vi "Check Condition.vi"(8 "error in (no error)":errorcluster, 11 "InterlockControl in":refnum<class "InterlockControl.lvclass">) -> (0 "error out":errorcluster, 2 "Interlocked":bool, 3 "InterlockControl out":refnum<class "InterlockControl.lvclass">)   [LabVIEW 2020, in "VolatusControl.lvlib" / "InterlockControl.lvclass"]
uses:
  InterlockControl.lvclass
  InterlockControl.lvclass/InterlockControl.ctl
  lv-vecto/Vecto/Channel DBL/Channel DBL.lvclass
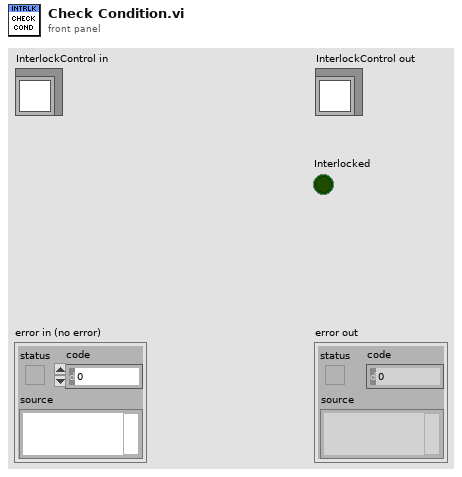
[diagram p1: front panel]
types:
  T1 = typedef "VolatusControl.lvlib/InterlockControl.lvclass/Inhibit Condition.ctl" = cluster{"Channel Name":string, "Comparison":T2, "Value":dbl}
  T2 = typedef "VolatusControl.lvlib/InterlockControl.lvclass/Inhibit Comparison.ctl" = enum16{"Equal", "Less Than", "Greater Than"}
  T3 = typedef "VolatusControl.lvlib/InterlockControl.lvclass/Inhibit Logic.ctl" = enum16{"Any", "All"}
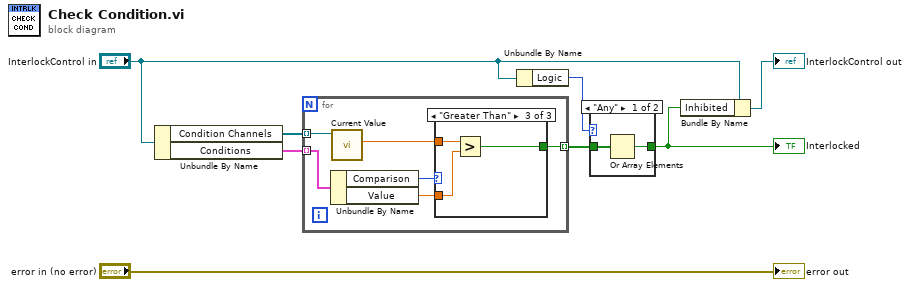
[diagram p0: block diagram]
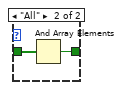
[diagram p2: hidden frame]
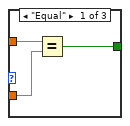
[diagram p3: hidden frame]
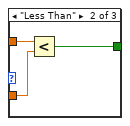
[diagram p4: hidden frame]
diagram:
  n1 = Unbundle By Name("InterlockControl in") -> ("Condition Channels"=w6:refnum<class "Channel DBL.lvclass">[], "Conditions"=w7:T1[])
  n2 = for {
    tunnel: w7 -> [w14] mode=indexing
    tunnel: w6 -> [w10] mode=indexing
    tunnel: [w9] -> w4 mode=indexing
    n3 = Unbundle By Name(w14) -> ("Comparison"=w13:T2, "Value"=w12:dbl)
    n4 = call "Current Value.vi"("Channel in"=w10) -> ("Scaled"=w11:dbl)  [unwired: 6 in, 4 out]
    n5 = case shown="\"Greater Than\"" w13 {
      tunnel: w12 -> [w16 w19 w22]
      tunnel: w11 -> [w17 w20 w23]
      tunnel: [w15 w18 w21] -> w9
      frame "Equal" {
        n6 = Equal?(x=w17, y=w16) -> (x = y?=w15:bool)
      }
      frame "Less Than" {
        n7 = Less?(x=w20, y=w19) -> (x < y?=w18:bool)
      }
      frame "Greater Than" {
        n8 = Greater?(x=w23, y=w22) -> (0:w21:bool)
      }
    }
  }
  n9 = Unbundle By Name("InterlockControl in") -> ("Logic"=w3:T3)
  n10 = case shown="\"Any\"" w3 {
    tunnel: w4 -> [w25 w27]
    tunnel: [w24 w26] -> w1
    frame "Any" {
      n11 = Or Array Elements(Boolean array=w25) -> (logical OR=w24:bool)
    }
    frame "All" {
      n12 = And Array Elements(Boolean array=w27) -> (logical AND=w26:bool)
    }
  }
  "Interlocked" <- w1
  n13 = Bundle By Name(cluster="InterlockControl in", "Inhibited"=w1) -> (→"InterlockControl out":refnum<class "InterlockControl.lvclass">)
  "error out" <- "error in (no error)"
